vi "Read Plugin Details.vi"(8 "error in (no error)":errorcluster, 10 "Plugin Details in":T2, 11 "Plugin File Refnum in":T1) -> (0 "error out":errorcluster, 2 "Plugin Details out":T2, 3 "Plugin File Refnum out":T1)   [LabVIEW 2020, in "RxnRover.lvlib" / "Plugin Manager.lvlib"]
uses:
  Plugin Manager.lvlib
  Plugin Details.ctl
  Plugin Servers/Controller/Controller Type.ctl
  Plugin Types.ctl
  Config Error.ctl
  <vilib>/Utility/config.llb/Config Data RefNum.ctl
  <vilib>/Utility/config.llb/Read Key (String).vi
  <vilib>/Utility/config.llb/NI_LVConfig.lvlib
  Plugin Servers/Controller/Generic Plugin.lvclass
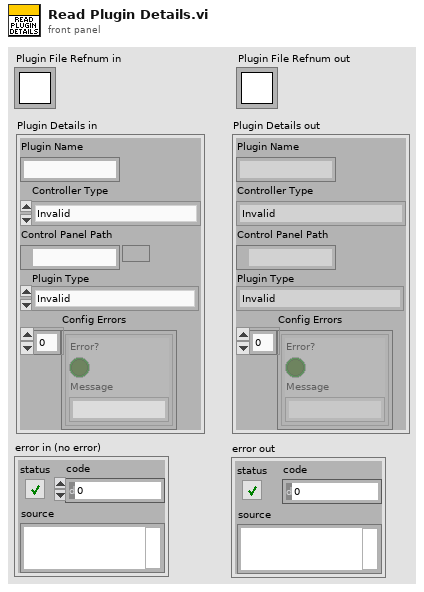
[diagram p1: front panel]
types:
  T1 = typedef "NI_LVConfig.lvlib/Config Data RefNum.ctl" = refnum<k1>
  T2 = typedef "RxnRover.lvlib/Plugin Manager.lvlib/Plugin Details.ctl" = cluster{"Plugin Name":string, "Controller Type":T3, "Control Panel Path":path, "Plugin Type":T4, "Config Errors":T5[]}
  T3 = typedef "RxnRover.lvlib/Generic Plugin.lvclass/Controller Type.ctl" = enum16{"Invalid", "Temperature Controller", "Pump Controller", "Syringe Pump", "Generic Optimizer", "LC Parser"}
  T4 = typedef "RxnRover.lvlib/Plugin Manager.lvlib/Plugin Types.ctl" = enum16{"Invalid", "Optimizer", "Analyzer", "Hardware"}
  T5 = typedef "RxnRover.lvlib/Plugin Manager.lvlib/Config Error.ctl" = cluster{"Error?":bool, "Message":string}
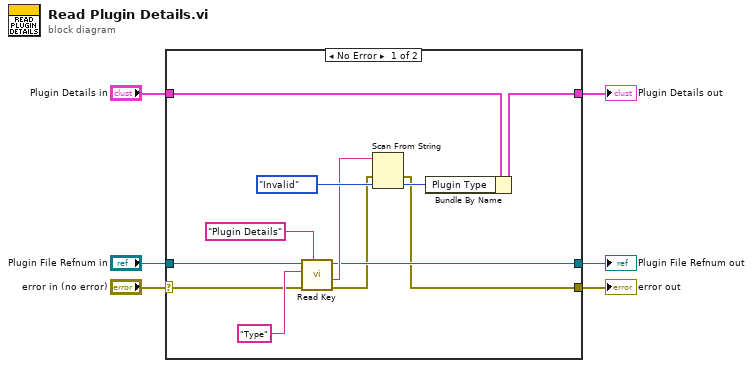
[diagram p0: block diagram]
diagram:
  n1 = case shown="No Error" "error in (no error)" {
    selector: "error in (no error)" -> [w9 w19]
    tunnel: [w15 w21] -> w6
    tunnel: "Plugin Details in" -> [w14 w21]
    tunnel: [w11 w20] -> w4
    tunnel: "Plugin File Refnum in" -> [w10 w20]
    tunnel: [w7 w19] -> w2
    frame No Error {
      n2 = call-poly <vilib>:"Read Key.vi"("section"="Plugin Details", "error in (no error)"=w9, "key"="Type", "refnum"=w10) -> ("error out"=w8:errorcluster, "value"=w16:string, "refnum out"=w11:T1)  [unwired: 4 in, 1 out]
      n3 = Scan From String(input string=w16, error in=w8, default 1=Plugin_Types."Invalid" ("Plugin Type")) -> (error out=w7:errorcluster, output 1=w18:T4)  [unwired: 2 in, 2 out]
      n4 = Bundle By Name(cluster=w14, "Plugin Type"=w18) -> (w15:T2)
    }
    frame Error {
    }
  }
  "Plugin Details out" <- w6
  "Plugin File Refnum out" <- w4
  "error out" <- w2
